vi "dfd_Build XML String.vi"(6 "add enter after the xml string":bool=TRUE, 7 "indent order":i32, 9 "string in":string, 11 "element name":string) -> (3 "xml string out":string)   [LabVIEW 2017, in "NI_DigFilter_Process.lvlib"]
uses:
  <vilib>/addons/Digital Filter Design/NI_DigFilter_Process.lvlib
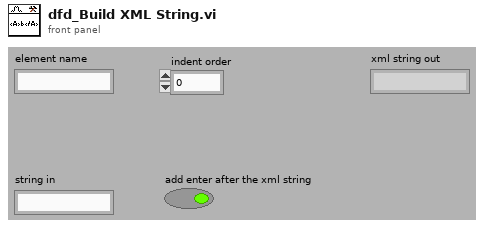
[diagram p1: front panel]
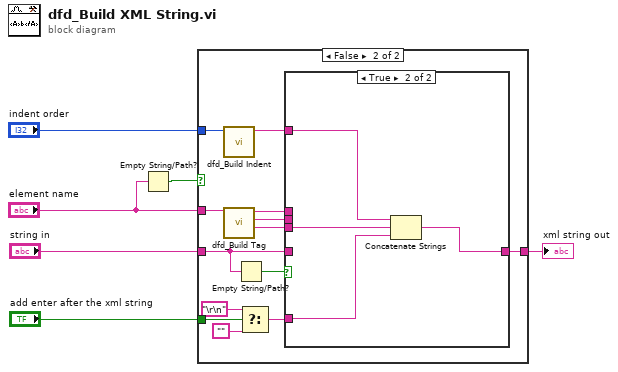
[diagram p0: block diagram]
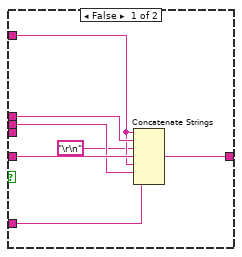
[diagram p3: hidden frame]
diagram:
  n1 = Empty String/Path?(string/path="element name") -> (empty?=w3:bool)
  n2 = case shown="False" w3 {
    tunnel: "element name" -> [_ w18]
    tunnel: [_ w19] -> w6
    tunnel: "string in" -> [_ w14]
    tunnel: "add enter after the xml string" -> [_ w10]
    tunnel: "indent order" -> [_ w7]
    frame True {
    }
    frame False {
      n3 = call <vilib>:"dfd_Build Indent.vi"("indent order"=w7) -> ("tag indent"=w12:string)  [unwired: 10 out]
      n4 = call <vilib>:"dfd_Build Tag.vi"("element name"=w18) -> ("empty tag"=w15:string, "end tag"=w16:string, "start tag"=w17:string)  [unwired: 8 out]
      n5 = Empty String/Path?(string/path=w14) -> (empty?=w13:bool)
      n6 = Select(t="\r\n", s=w10, f="") -> (s? t:f=w8:string)
      n7 = case shown="True" w13 {
        tunnel: [w26 w28] -> w19
        tunnel: w14 -> [w25 _]
        tunnel: w17 -> [w23 _]
        tunnel: w16 -> [w22 _]
        tunnel: w15 -> [_ w29]
        tunnel: w12 -> [w21 w30]
        tunnel: w8 -> [w24 w27]
        frame False {
          n8 = Concatenate Strings(w21, w23, "\r\n", w25, w21, w22, w24) -> (w26:string)
        }
        frame True {
          n9 = Concatenate Strings(w30, w29, w27) -> (w28:string)
        }
      }
    }
  }
  "xml string out" <- w6
